vi "Build Bulk Create.vi"(8 "error in (no error)":errorcluster, 9 "tableName":string, 10 "DynamicParameters in":refnum<class "DynamicParameters.lvclass">[](array[class]), 11 "PostgresqlConnection in":refnum<class "DBC.lvclass">) -> (0 "error out":errorcluster, 2 "BulkInsertQuery":string, 3 "PostgresqlConnection out":refnum<class "DBC.lvclass">)   [LabVIEW 2020, in "ORM_DBC_Npgsql.lvlib" / "DBC.lvclass"]
uses:
  DBC.lvclass
  <vilib>/Viviota/shared/ORM.lvlibp/ORM/DynamicParameters/DynamicParameters.lvclass
  <vilib>/Viviota/shared/ORM.lvlibp/ORM/DynamicParameters/Read AutoKey.vi
  <vilib>/Viviota/shared/ORM_DBC_dotNet.lvlibp/dbcDotNet/ORM_DBC_dotNet.lvclass
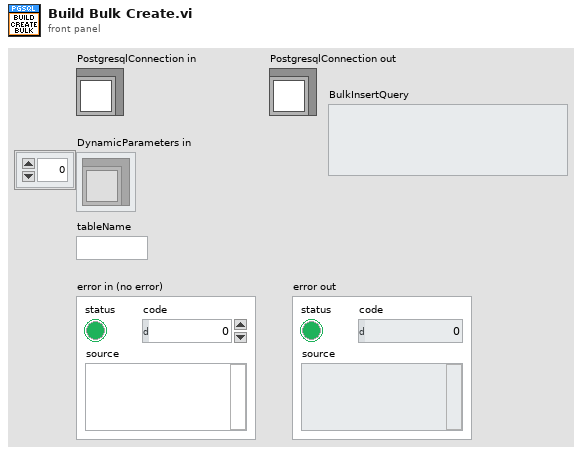
[diagram p1: front panel]
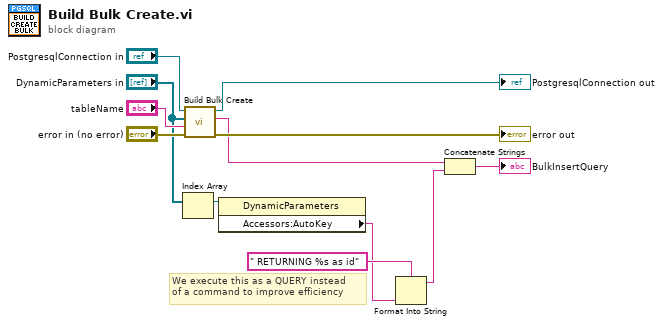
[diagram p0: block diagram]
diagram:
  # "We execute this as a QUERY instead\nof a command to improve efficiency"
  n1 = Index Array(array="DynamicParameters in") -> (element=w3:refnum<class "DynamicParameters.lvclass">)  [unwired: 1 in]
  n2 = call-parent "Build Bulk Create.vi"("error in (no error)"="error in (no error)", "tableName"="tableName", "DynamicParameters in"="DynamicParameters in", "DbConnection in"="PostgresqlConnection in") -> ("error out"=→"error out":errorcluster, "BulkInsertQuery"=w2:string, "DbConnection out"=→"PostgresqlConnection out":refnum<class "DBC.lvclass">)  [unwired: 5 in]
  n3 = property class="DynamicParameters"(reference=w3) -> ("Accessors:AutoKey"=w6:string)  [unwired: 1 in, 2 out]
  n4 = Format Into String(format string=" RETURNING %s as id" ("string"), w6) -> (resulting string=w5:string)  [unwired: 2 in, 1 out]
  n5 = Concatenate Strings(w2, w5) -> (→"BulkInsertQuery":string)
